vi "Run Service.vi"() -> ()   [LabVIEW 2019, in "route_guide_server.lvlib"]
uses:
  route_guide_server.lvlib
  RPC Service/RouteGuide/RouteGuide.lvclass
  C:/Program Files (x86)/National Instruments/LabVIEW 2019/vi.lib/gRPC/LabVIEW gRPC Servicer/ServiceBase/ServiceBase.lvclass
  <vilib>/gRPC/LabVIEW gRPC Servicer/Servicer/Servicer.lvclass/Servicer.ctl
  <vilib>/gRPC/LabVIEW gRPC Servicer/Servicer/Servicer.lvclass
  Is Call Cancelled Global.vi
  Server Error Global.vi
panel:
  out "Server Error":errorcluster
  out "Is Call Cancelled?":bool
  out "Listening Port":i32
  in  "Stop":bool
  in  "Server Address":string="localhost:50051"
  in  "Server Certificate File (.crt)":path
  in  "Server Key File (.key)":path
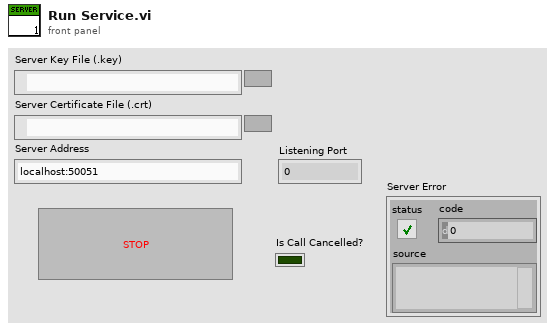
[diagram p1: front panel]
types:
  T1 = typedef "grpc-lvsupport-release.lvlib/grpcId.ctl" = u64
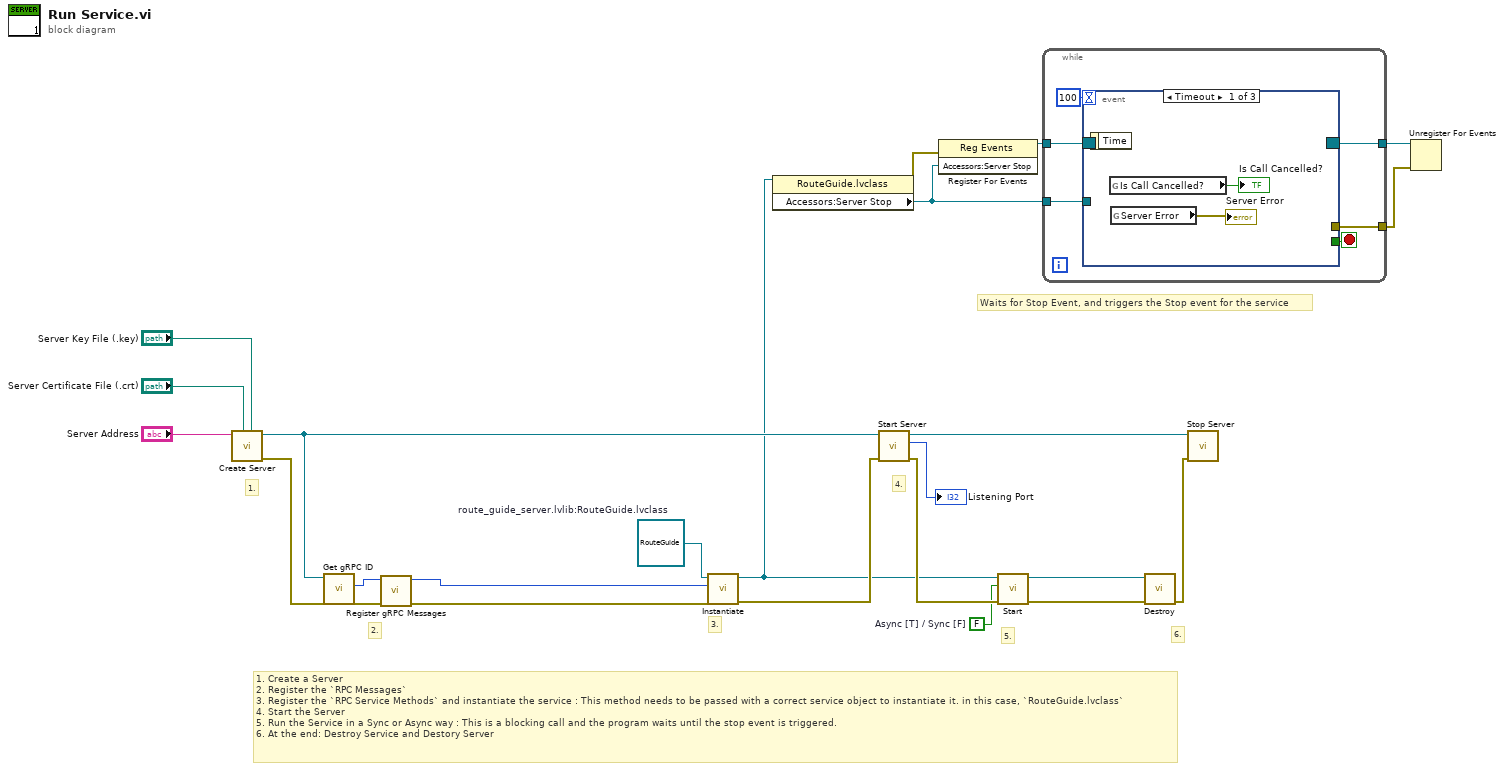
[diagram p0: block diagram]
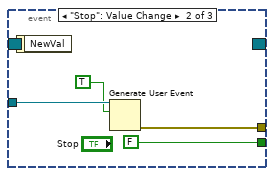
[diagram p2: hidden frame]
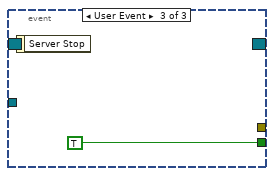
[diagram p3: hidden frame]
diagram:
  w4 = FALSE  # Async [T] / Sync [F]
  w1 = refnum<class "RouteGuide.lvclass"> refnum  # route_guide_server.lvlib:RouteGuide.lvclass
  # "Waits for Stop Event, and triggers the Stop event for the service"
  # "6."
  # "5."
  # "4."
  # "3."
  # "2."
  # "1."
  # "1. Create a Server\n2. Register the `RPC Messages`\n3. Register the `RPC Service Methods` and instantiate the service : This method needs to be passed with a correct service object to instantiate it. in this case, `RouteGuide.lvclass`\n4. Start the Server\n5. Run the Service in a Sync or Async way : This is a blocking call and the program waits until the stop event is triggered.\n6. At the end: Destroy Service and Destory Server"
  n1 = call <vilib>:"Create Server.vi"("Server Key File (.key)"="Server Key File (.key)", "Server Certificate File (.crt)"="Server Certificate File (.crt)", "Server Address"="Server Address") -> ("error out"=w10:errorcluster, "gRPC Server out"=w16:refnum<class "Servicer.lvclass">)  [unwired: 7 in]
  n2 = call <vilib>:"Get gRPC ID.vi"("OOP Server in"=w16) -> ("gRPC ID"=w11:T1)  [unwired: 9 in, 1 out]
  n3 = call "Register gRPC Messages.vi"("error in (no error)"=w10, "gRPC ID"=w11) -> ("error out"=w9:errorcluster, "gRPC ID Out"=w8:T1)  [unwired: 8 in]
  n4 = call-dynamic "Instantiate.vi"("error in"=w9, "gRPCid"=w8, "iService"=w1) -> ("error out"=w14:errorcluster, "iService"=w3:refnum<class "RouteGuide.lvclass">)  [unwired: 7 in]
  n5 = property class="RouteGuide.lvclass"(reference=w3) -> (error out=w15:errorcluster, "Accessors:Server Stop"=w2:refnum<user-event>)  [unwired: 1 in, 1 out]
  n6 = call <vilib>:"Start Server.vi"("error in"=w14, "gRPC Server in"=w16) -> ("error out"=w7:errorcluster, "Listening Port"=→"Listening Port":i32, "gRPC Server out"=w23:refnum<class "Servicer.lvclass">)  [unwired: 7 in]
  n7 = register-events(error in=w15, w2) -> (reference out=w19:refnum<event-registration>)  [unwired: 1 in, 1 out]
  n8 = call-dynamic "Start.vi"("error in"=w7, "ASync [T]"=w4, "iService in"=w3) -> ("error out"=w6:errorcluster, "iService out"=w5:refnum<class "RouteGuide.lvclass">)  [unwired: 7 in]
  n9 = while {
    tunnel: w19 -> [w29]
    tunnel: [w27] -> w18
    tunnel: [w25] -> w12
    tunnel: w2 -> [w26]
    stop <- w28 stop-if-true
    n10 = event shown="[0] Timeout" {
      selector: w29 -> [_ _ _]
      dyn-events: [_ _ _] -> w27
      timeout: 100 -> [_ _ _]
      tunnel: [_ FALSE TRUE] -> w28
      tunnel: w26 -> [_ w34 _]
      tunnel: [_ w32 _] -> w25
      event Timeout {
        n11 = event-data() -> ()  [unwired: 1 in, 1 out]
        n12 = global read "Is Call Cancelled Global.vi" "Is Call Cancelled?"() -> (→"Is Call Cancelled?":bool)
        n13 = global read "Server Error Global.vi" "Server Error"() -> (→"Server Error":errorcluster)
      }
      event "Stop": Value Change {
        n14 = event-data() -> ()  [unwired: 1 in, 1 out]
        n15 = Generate User Event(user event=w34, event data cluster=TRUE ("event data")) -> (error out=w32:errorcluster)  [unwired: 2 in, 1 out]
      }
      event User Event {
        n16 = event-data() -> ()  [unwired: 1 in, 1 out]
      }
    }
  }
  n17 = call-dynamic "Destroy.vi"("error in (no error)"=w6, "SignalGeneratorService in"=w5) -> ("error out"=w13:errorcluster)  [unwired: 8 in, 1 out]
  n18 = call <vilib>:"Stop Server.vi"("error in"=w13, "gRPC Server in"=w23) -> ()  [unwired: 9 in, 1 out]
  n19 = Unregister For Events(event registration refnum=w18, error in=w12) -> ()  [unwired: 1 out]
